vi "CLD 17 GUI number pad solution.vi"(8 "error in (no error)":errorcluster) -> (0 "error out":errorcluster, 3 "Numeric":dbl)   [LabVIEW 2009]
doc: "CLD 17 Exercise\n\nThis VI uses a polling method to respond to changes in the GUI. The key index is based on the tabbing order of the control type def. An action selector case is provided for future expansion for back space."
uses:
  CLD 17 Keypad_Typedef.ctl
panel:
  out "String":string
  in  "Keypad Cluster":T1
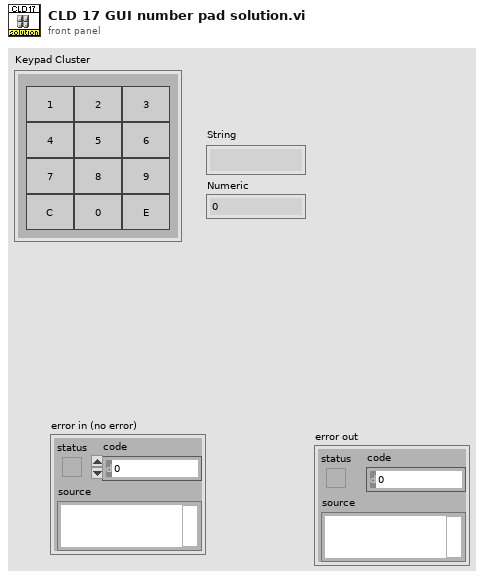
[diagram p1: front panel]
types:
  T1 = typedef "CLD 17 Keypad_Typedef.ctl" = cluster{"0":bool, "1":bool, "2":bool, "3":bool, "4":bool, "5":bool, "6":bool, "7":bool, "8":bool, "9":bool, "C":bool, "E":bool}
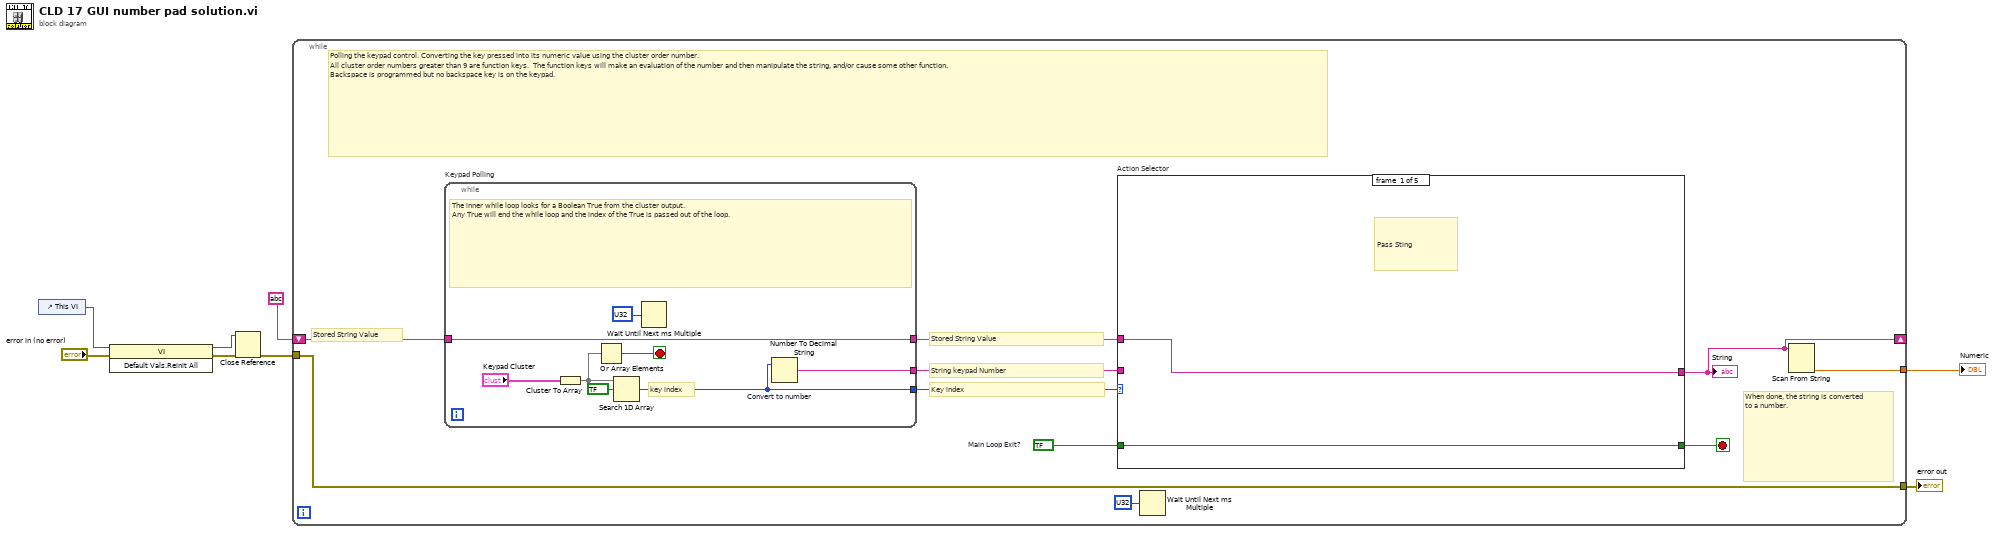
[diagram p0: block diagram]
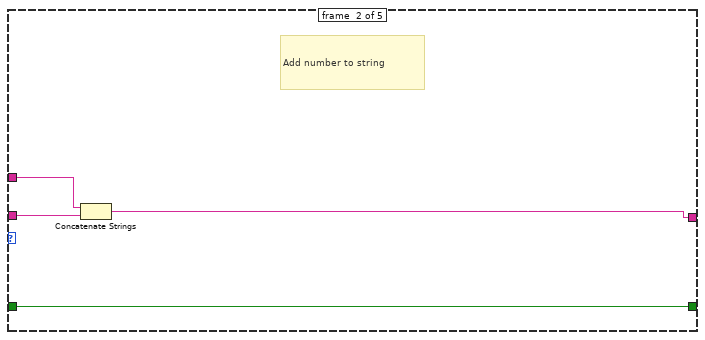
[diagram p2: hidden frame]
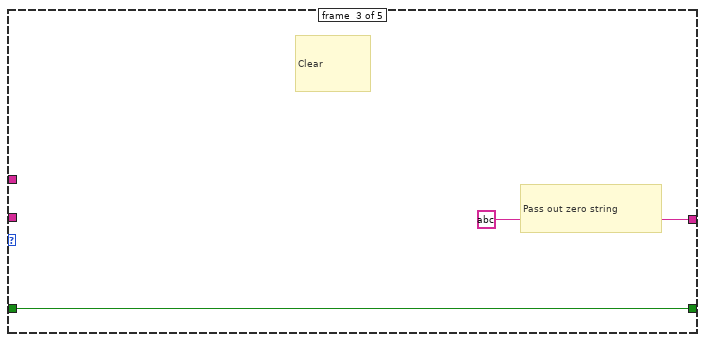
[diagram p3: hidden frame]
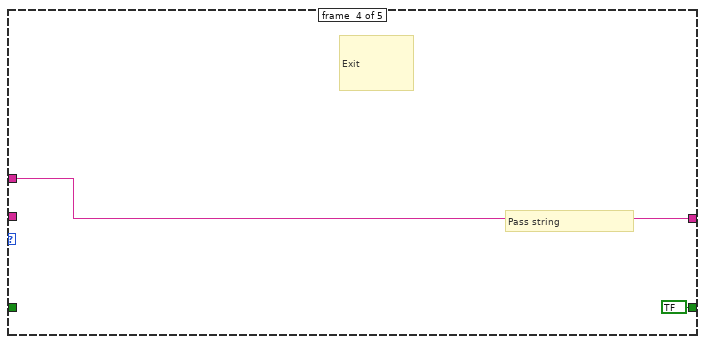
[diagram p4: hidden frame]
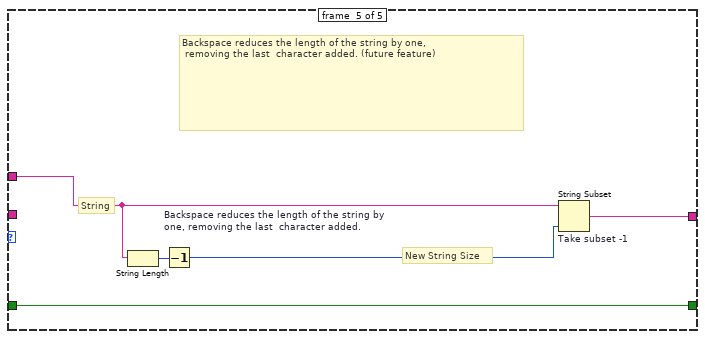
[diagram p5: hidden frame]
diagram:
  n1 = control-ref of="This VI"() -> (w7:refnum<vi>)
  n2 = invoke class="VI" method="Default Vals.Reinit All"(reference=w7, error in="error in (no error)") -> (reference out=w4:refnum<vi>, error out=w6:errorcluster)  [unwired: 1 in, 1 out]
  n3 = Close Reference(reference=w4, error in (no error)=w6) -> (error out=w5:errorcluster)
  n4 = while {
    shift-right: [w14] -> _
    shift-left: string ? -> [w11]
    tunnel: w5 -> [w9]
    tunnel: [w18] -> w3
    tunnel: [w9] -> w1
    stop <- w13 stop-if-true
    w12 = bool ?  # Main Loop Exit?
    # "When done, the string is converted to a number."
    # "Polling the keypad control. Converting the key pressed into its numeric value using the cluster order number. \nAll cluster order numbers greater than 9 are function keys.  The function keys will make an evaluation of the number and then manipulate the string, and/or cause some other function.  \nBackspace is programmed but no backspace key is on the keypad."
    # "Key index"
    # "String keypad Number"
    # "Stored String Value"
    # "Stored String Value"
    n5 = while "Keypad Polling" {
      tunnel: [w36] -> w16
      tunnel: [w35] -> w15
      tunnel: [w34] -> w10
      tunnel: w11 -> [w34]
      stop <- w38 stop-if-true
      # "key index"
      # "The inner while loop looks for a Boolean True from the cluster output.\nAny True will end the while loop and the index of the True is passed out of the loop."
      n6 = Cluster To Array(cluster="Keypad Cluster") -> (array=w39:bool[])
      n7 = Or Array Elements(Boolean array=w39) -> (logical OR=w38:bool)
      n8 = Search 1D Array(1D array=w39, element=bool ?) -> (index of element=w36:i32)  [unwired: 1 in]
      n9 = Wait Until Next ms Multiple(millisecond multiple=u32 ?) -> ()  [unwired: 1 out]
      n10 = Number To Decimal String "Convert to number"(number=w36) -> (decimal integer string=w35:string)  [unwired: 1 in]
    }
    n11 = case "Action Selector" shown="10" w16 {
      tunnel: w10 -> [w20 w24 _ w28 w30]
      tunnel: w15 -> [_ w23 _ _ _]
      tunnel: [w20 w22 string ? w28 w31] -> w14
      tunnel: [w19 w21 w26 bool ? w29] -> w13
      tunnel: w12 -> [w19 w21 w26 _ w29]
      frame #0 {
        # "Pass Sting"
      }
      frame #1 {
        # "Add number to string"
        n12 = Concatenate Strings(w24, w23) -> (w22:string)
      }
      frame #2 {
        # "Pass out zero string"
        # "Clear"
      }
      frame #3 {
        # "Pass string"
        # "Exit"
      }
      frame #4 {
        # "New String Size"
        # "String"
        # "Backspace reduces the length of the string by one,\n removing the last  character added. (future feature)"
        n13 = String Length(string=w30) -> (length=w33:i32)
        n14 = Decrement "Backspace reduces the length of the string by one, removing the last  character added."(x=w33) -> (x-1=w32:i32)
        n15 = String Subset "Take subset -1"(string=w30, length (rest)=w32) -> (substring=w31:string)  [unwired: 1 in]
      }
    }
    "String" <- w14
    n16 = Wait Until Next ms Multiple(millisecond multiple=u32 ?) -> ()  [unwired: 1 out]
    n17 = Scan From String(input string=w14) -> (output 1=w18:dbl)  [unwired: 4 in, 3 out]
  }
  "Numeric" <- w3
  "error out" <- w1
